vi "清空数据左右.vi"(11 "数组输入":string[](array[string])) -> (3 "数组输出":string[](array[string]))   [LabVIEW 2011]
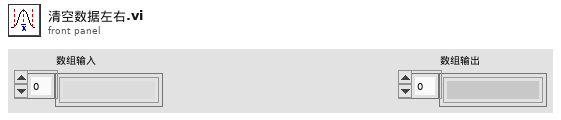
[diagram p1: front panel]
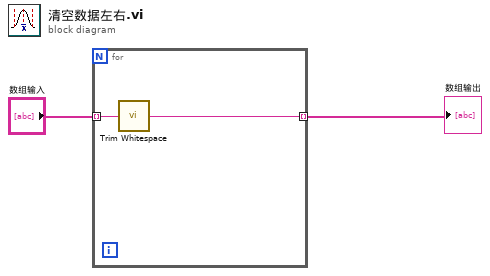
[diagram p0: block diagram]
diagram:
  n1 = for {
    tunnel: "数组输入" -> [w4] mode=indexing
    tunnel: [w3] -> w1 mode=indexing
    n2 = call <vilib>:"Trim Whitespace.vi"("string"=w4) -> ("trimmed string"=w3:string)  [unwired: 1 in]
  }
  "数组输出" <- w1
